vi "Escribir_propiedades.vi"() -> ()   [LabVIEW 2016]
panel:
  in  "Stop Button":bool
  out "Boolean":bool
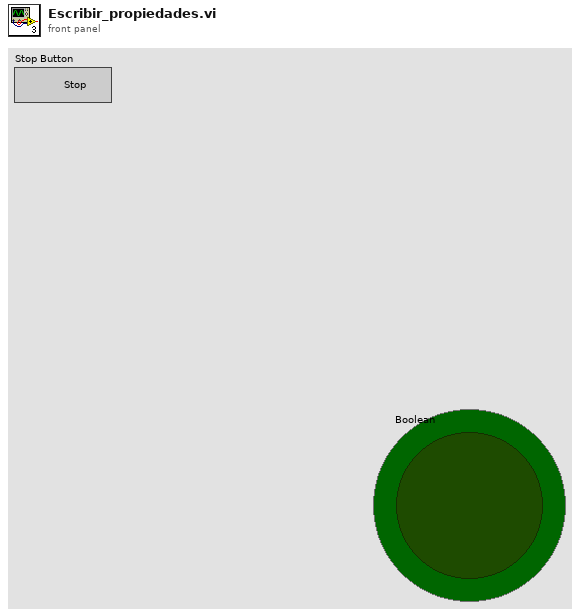
[diagram p1: front panel]
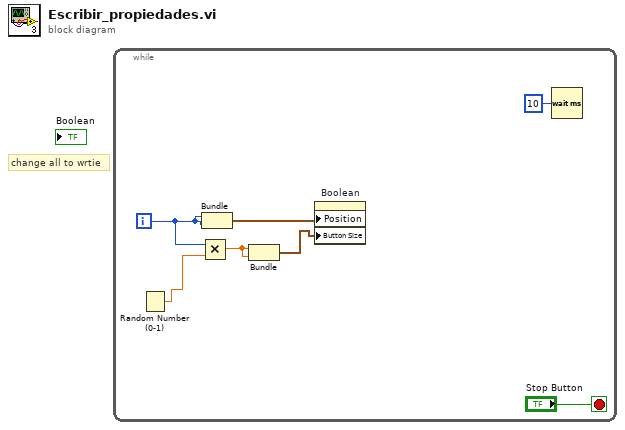
[diagram p0: block diagram]
diagram:
  # "change all to wrtie"
  n1 = while {
    i -> [w4]
    stop <- "Stop Button" stop-if-true
    n2 = Random Number (0-1)() -> (number: 0 to 1=w3:dbl)
    n3 = Multiply(x=w4, y=w3) -> (x*y=w2:dbl)
    n4 = Bundle(w4, w4) -> (w6:cluster{i32, i32})  [unwired: 1 in]
    n5 = Bundle(w2, w2) -> (w1:cluster{dbl, dbl})  [unwired: 1 in]
    n6 = property on="Boolean" class="Bool (strict)"("Position"=w6, "Button Size"=w1) -> ()  [unwired: 2 in, 2 out]
    n7 = Wait (ms)(milliseconds to wait=u32 10) -> ()  [unwired: 1 out]
  }
